vi "MainNR.vi"(10 "JQMHStartup":refnum<class "RQMHStartup.lvclass">, 11 "NewTemplate in":refnum<class "Shell.lvclass">) -> ()   [LabVIEW 2024, in "Shell.lvclass"]
uses:
  Shell.lvclass
  RQMHCore/Startup/RQMHStartup.lvclass
  RQMHCore/ModQueue/RQMHMessageQueue.lvclass/RQMHMessageQueue.ctl
  RQMHCore/ModuleCore/InitialiseReplyArgs.ctl
  RQMHCore/ModuleCore/RQMHModule.lvclass/RQMHModule.ctl
  Do Something ReplyArgs.ctl
  Do Something Args.ctl
  GetContents ReplyArgs.ctl
  Maximise Args.ctl
  RQMHCore/ModuleCore/Read ModuleName.vi
  RQMHCore/ModuleCore/Read External Start.vi
  RQMHCore/ModQueue/Delacor_lib_QMH_Enqueue Message (Single).vi
  RQMHCore/ModQueue/RQMHMessageQueue.lvclass
  RQMHCore/ModuleCore/RQMHModule.lvclass
  RQMHCore/Shared/RQMHShared.lvlib
panel:
  out "error out":errorcluster
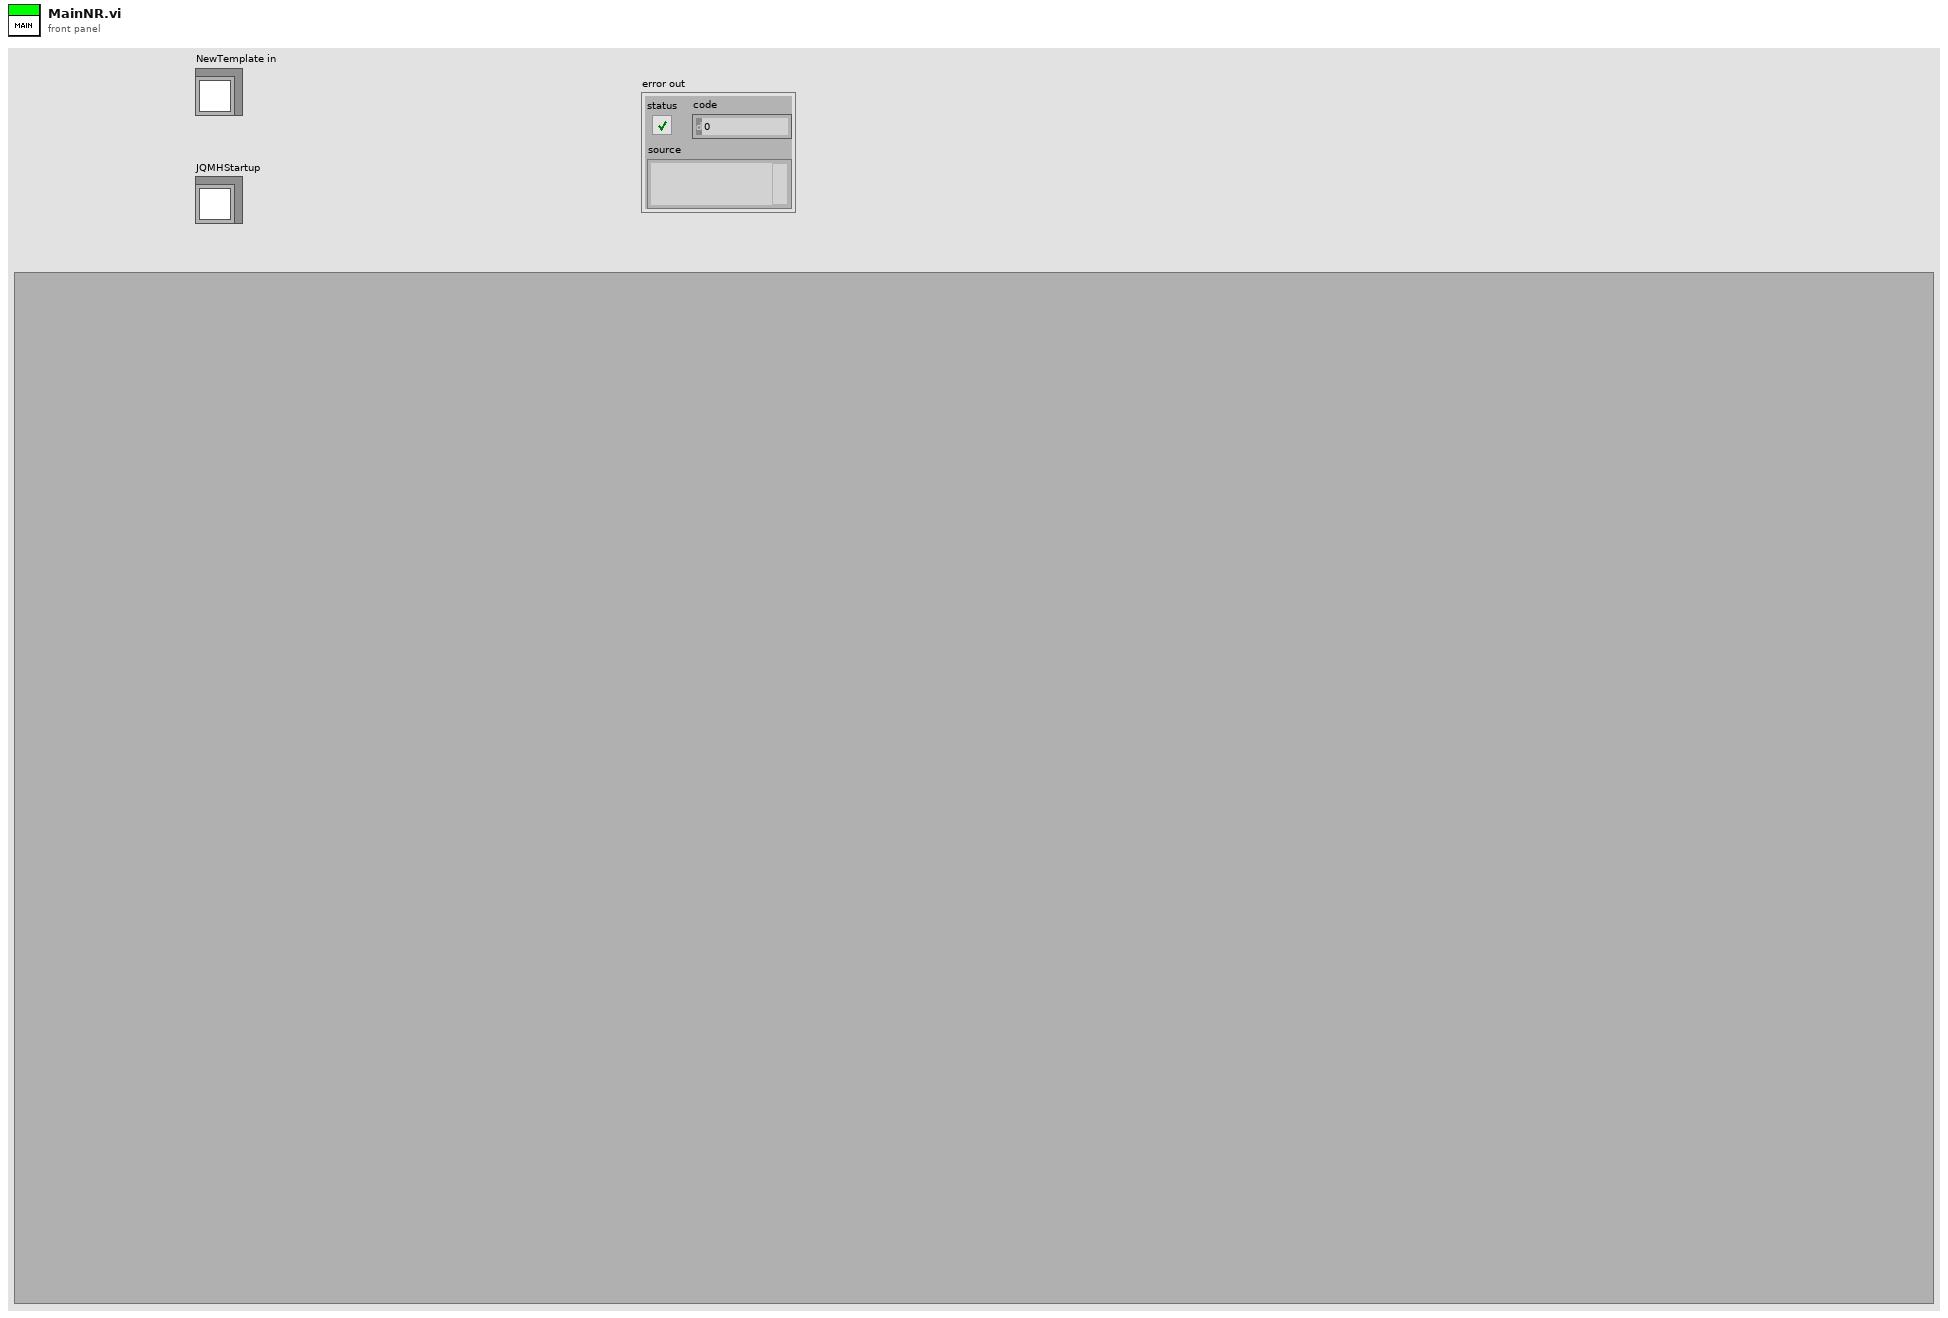
[diagram p1: front panel]
types:
  T1 = typedef "Shell.lvclass/Request Events--cluster.ctl" = cluster{"Do Something":refnum<user-event>, "GetContents":refnum<user-event>, "Maximise":refnum<user-event>, "Minimise":refnum<user-event>}
  T2 = cluster{"Stop Module":refnum<user-event>, "Requests":T1}
  T3 = enum32{"Invalid", "Standard", "Closed", "Hidden", "Minimized", "Maximized"}
  T4 = typedef "RQMHModule.lvclass/InitialiseReplyArgs.ctl" = cluster{"Did Init?":bool}
  T5 = typedef "Shell.lvclass/Do Something Args.ctl" = cluster{"Msg":string}
  T6 = typedef "Shell.lvclass/Do Something ReplyArgs.ctl" = cluster{"Value":dbl, "Boolean":bool}
  T7 = typedef "Shell.lvclass/GetContents ReplyArgs.ctl" = cluster{"Sub Panel":refnum<vi>}
  T8 = typedef "Shell.lvclass/Maximise Args.ctl" = cluster{"Maximise":bool}
  T9 = typedef "RQMHModule.lvclass/Reply.ctl" = cluster{"Expects Reply":bool, "Reply":refnum<notifier>}
  T10 = typedef "Shell.lvclass/GetContents Args.ctl" = cluster{"String":string}
  T11 = typedef "Shell.lvclass/Minimise Args.ctl" = cluster{"null":bool}
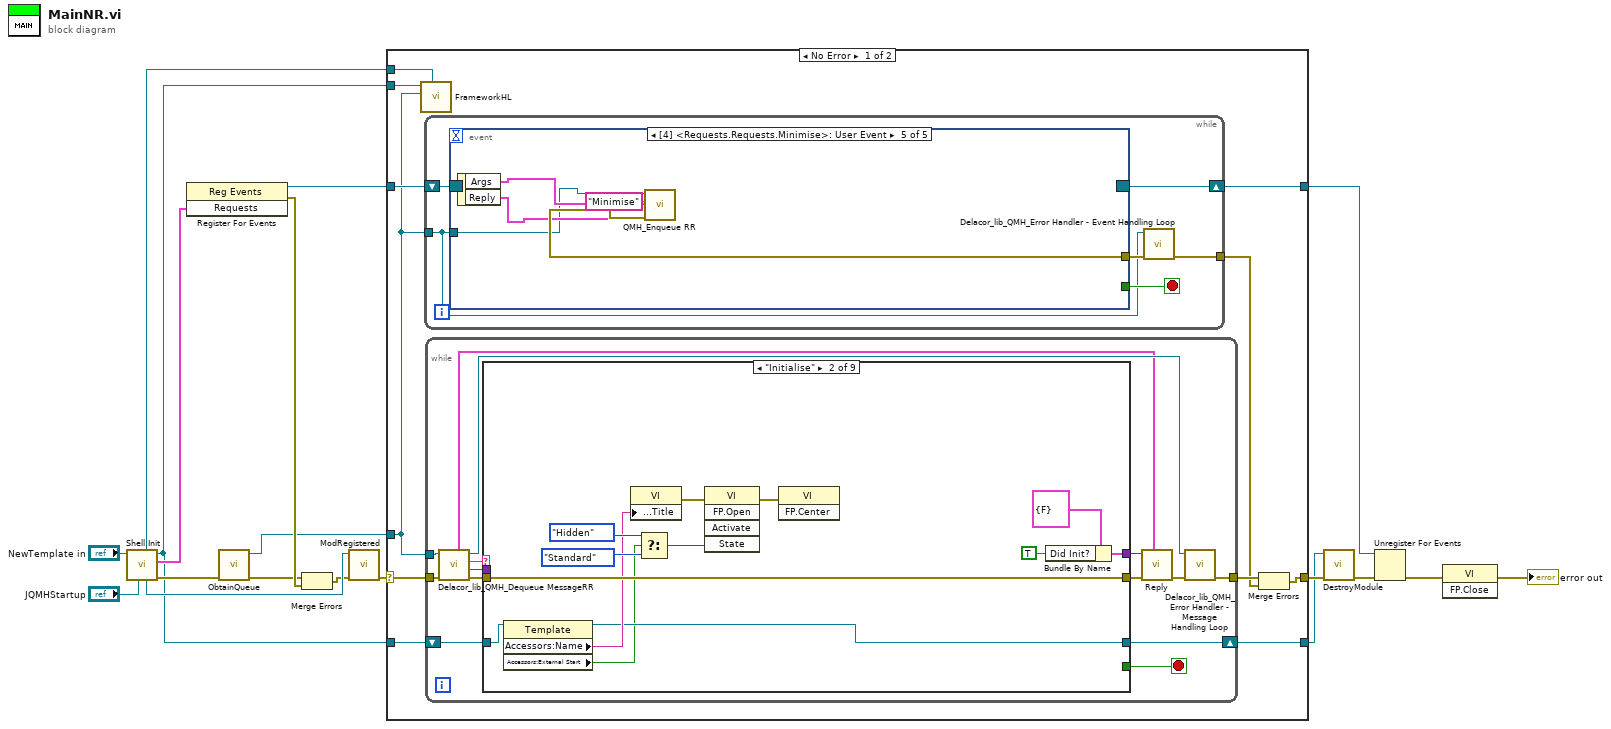
[diagram p0: block diagram]
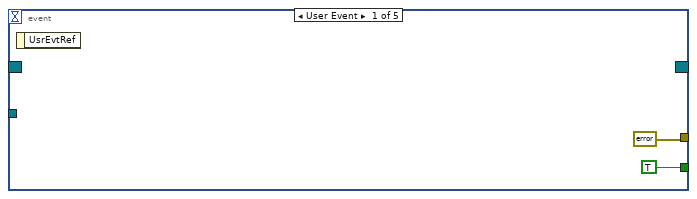
[diagram p2: hidden frame]
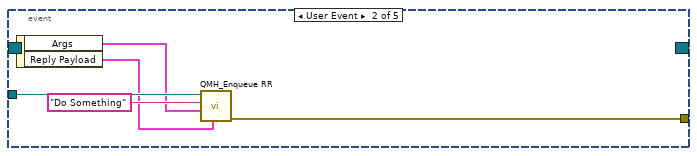
[diagram p3: hidden frame]
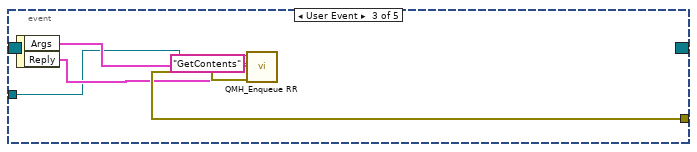
[diagram p4: hidden frame]
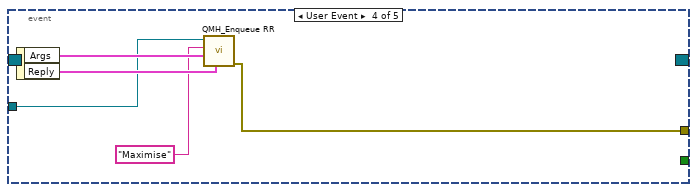
[diagram p5: hidden frame]
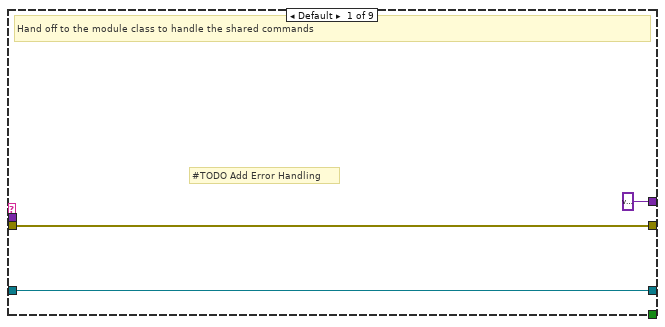
[diagram p6: hidden frame]
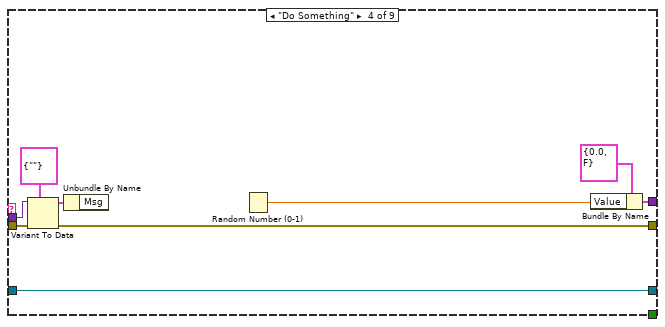
[diagram p8: hidden frame]
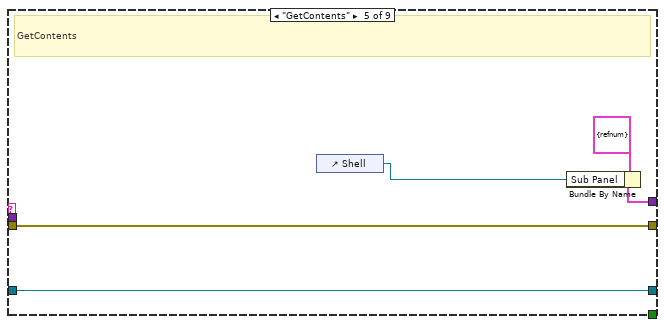
[diagram p9: hidden frame]
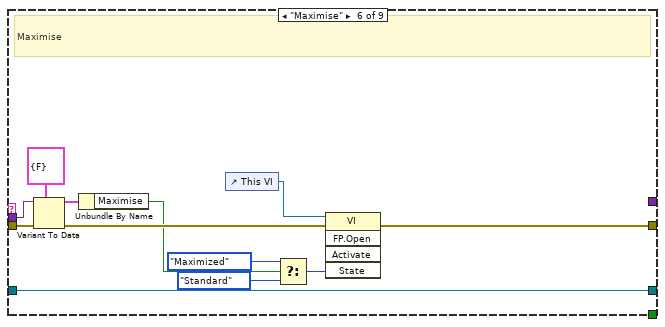
[diagram p10: hidden frame]
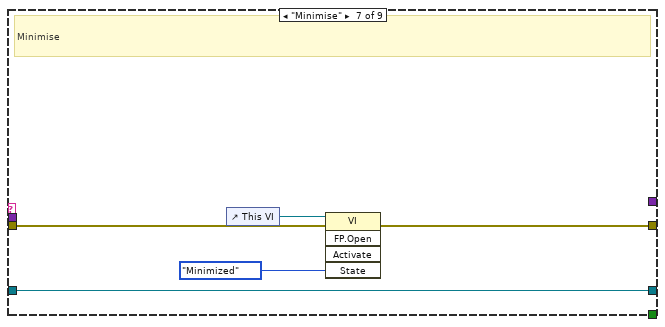
[diagram p11: hidden frame]
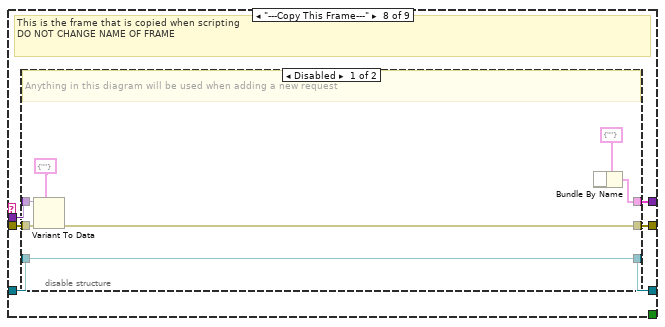
[diagram p12: hidden frame]
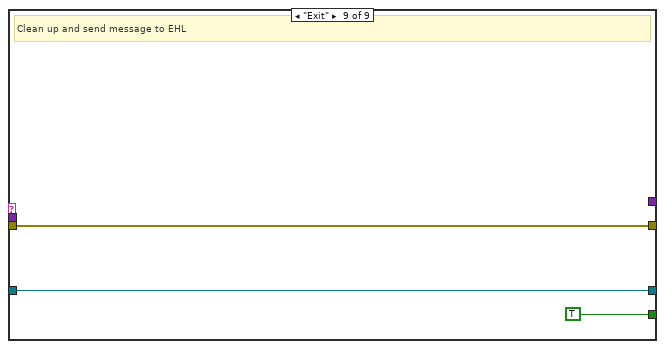
[diagram p14: hidden frame]
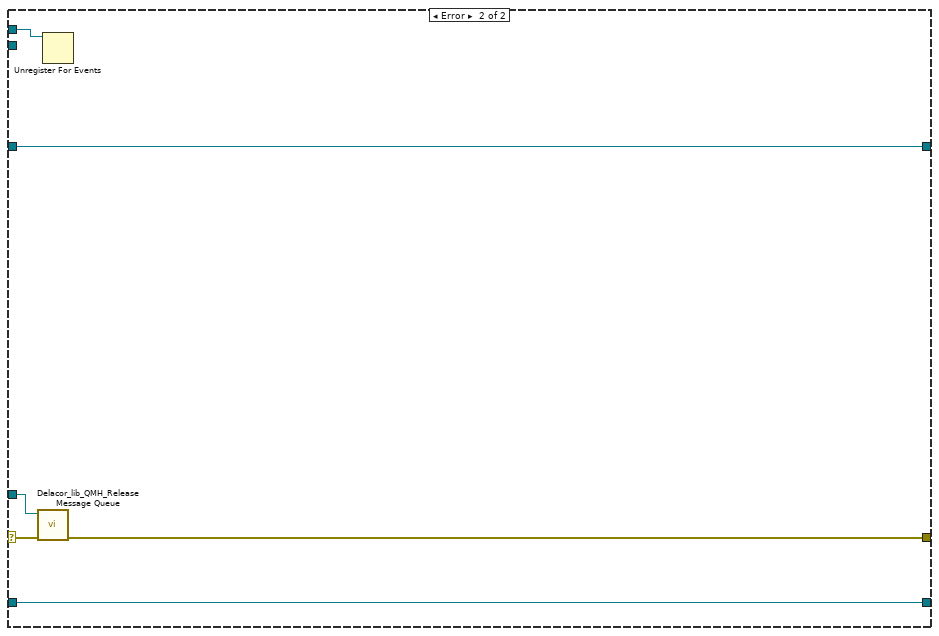
[diagram p15: hidden frame]
diagram:
  n1 = call "Shell.Init.vi"("JQMHStartup in"="JQMHStartup", "NewTemplate in"="NewTemplate in") -> ("error out"=w13:errorcluster, "Requests"=w4:T2, "NewTemplate out"=w3:refnum<class "Shell.lvclass">, "JQMHStartup out"=w11:refnum<class "RQMHStartup.lvclass">, "StandardRequests"=w7:refnum<event-registration>)  [unwired: 4 in, 1 out]
  n2 = register-events(w4) -> (reference out=w6:refnum<event-registration>, error out=w19:errorcluster)  [unwired: 2 in]
  n3 = call "ObtainQueue.vi"("error in"=w13) -> ("error out"=w12:errorcluster, "Message Queue"=w8:refnum<class "RQMHMessageQueue.lvclass">)  [unwired: 9 in]
  n4 = Merge Errors(w12, w19) -> (w9:errorcluster)
  n5 = call "ModRegistered.vi"("error in (no error)"=w9, "JQMHStartup in"=w11) -> ("error out"=w10:errorcluster)  [unwired: 9 in]
  n6 = case "RQMH_MAIN" shown="No Error" w10 {
    selector: w10 -> [w27 w143]
    tunnel: w3 -> [w30 w142]
    tunnel: [w29 w145] -> w18
    tunnel: w6 -> [w28 w145]
    tunnel: w8 -> [w21 w144]
    tunnel: [w26 w142] -> w5
    tunnel: [w23 w141] -> w15
    tunnel: w3 -> [w22 _]
    tunnel: w7 -> [w20 w140]
    frame No Error {
      n7 = call-dynamic "FrameworkHL.vi"("StandardRequests"=w20, "Message Queue"=w21, "JQMHModule in"=w22) -> ()  [unwired: 9 in]
      n8 = while {
        shift-right: [w36] -> w29
        shift-left: w28 -> [w31]
        tunnel: w21 -> [w32]
        tunnel: [w33] -> w24
        stop <- w35 stop-if-true
        n9 = event "RQMH_EVENT_MAIN" shown="[4] <Requests.Requests.Minimise>: User Event" {
          selector: w31 -> [_ _ _ _ _]
          dyn-events: [_ _ _ _ _] -> w36
          timeout: _ -> [_ _ _ _ _]
          tunnel: [TRUE _ _ _ _] -> w35
          tunnel: w32 -> [_ w43 w45 w50 w55]
          tunnel: [errorcluster {"status"=FALSE, "code"=0, "source"=""} ("error out") w40 w48 w53 w58] -> w34
          event User Event {
            n10 = event-data() -> ()  [unwired: 1 in, 1 out]
          }
          event User Event {
            n11 = event-data() -> ("Args"=w41:T5, "Reply Payload"=w39:T9)  [unwired: 1 in]
            n12 = call "QMH_Enqueue RR.vi"("Reply"=w39, "Message Data"=w41, "Message"="Do Something", "Message Queue in"=w43) -> ("error out"=w40:errorcluster)  [unwired: 6 in, 1 out]
          }
          event User Event {
            n13 = event-data() -> ("Args"=w46:T10, "Reply"=w47:T9)  [unwired: 1 in]
            n14 = call "QMH_Enqueue RR.vi"("Reply"=w47, "Message Data"=w46, "Message"="GetContents", "Message Queue in"=w45) -> ("error out"=w48:errorcluster)  [unwired: 6 in, 1 out]
          }
          event User Event {
            n15 = event-data() -> ("Args"=w51:T8, "Reply"=w52:T9)  [unwired: 1 in]
            n16 = call "QMH_Enqueue RR.vi"("Reply"=w52, "Message Data"=w51, "Message"="Maximise", "Message Queue in"=w50) -> ("error out"=w53:errorcluster)  [unwired: 6 in, 1 out]
          }
          event User Event {
            n17 = event-data() -> ("Args"=w56:T11, "Reply"=w57:T9)  [unwired: 1 in]
            n18 = call "QMH_Enqueue RR.vi"("Reply"=w57, "Message Data"=w56, "Message"="Minimise", "Message Queue in"=w55) -> ("error out"=w58:errorcluster)  [unwired: 6 in, 1 out]
          }
        }
        n19 = call-dynamic "Delacor_lib_QMH_Error Handler - Event Handling Loop.vi"("error in"=w34, "Message Queue in"=w32) -> ("dup error in"=w33:errorcluster)  [unwired: 8 in, 1 out]
      }
      n20 = while {
        tunnel: w21 -> [w67]
        tunnel: w27 -> [w66]
        shift-right: [w69] -> w26
        shift-left: w30 -> [w70]
        tunnel: [w68] -> w25
        stop <- w72 stop-if-true
        n21 = call-dynamic "Delacor_lib_QMH_Dequeue MessageRR.vi"("error in"=w66, "Message Queue in"=w67) -> ("error out"=w65:errorcluster, "Message Data"=w63:variant, "Message"=w64:string, "Message Queue out"=w71:refnum<class "RQMHMessageQueue.lvclass">, "Reply"=w59:T9)  [unwired: 5 in]
        n22 = case "RQMH_MESSAGE_CASES" shown="\"Initialise\"" w64 {
          tunnel: [_ _ _ _ _ _ _ _ TRUE] -> w72
          tunnel: w70 -> [w74 w77 w89 w99 w103 w115 w121 w125 w138]
          tunnel: w63 -> [_ _ _ w95 _ w114 _ w123 _]
          tunnel: w65 -> [w75 w88 w90 w94 w104 w116 w119 w127 w137]
          tunnel: [w75 w88 w90 w93 w104 w109 w118 w126 w137] -> w62
          tunnel: [w74 w78 w89 w99 w103 w115 w121 w124 w138] -> w69
          tunnel: [variant w87 _ w98 w102 _ _ w122 _] -> w60
          frame Default {
            # "#TODO Add Error Handling"
            # "Hand off to the module class to handle the shared commands"
          }
          frame "Initialise" {
            n23 = property class="Template"(reference=w77) -> (reference out=w78:refnum<class "Shell.lvclass">, "Accessors:Name"=w79:string, "Accessors:External Start"=w76:bool)  [unwired: 1 in, 1 out]
            n24 = property on="Property Node" class="VI"("Front Panel.Title"=w79) -> (error out=w85:errorcluster)  [unwired: 2 in, 1 out]
            n25 = Select(t=T3."Hidden" ("State"), s=w76, f=T3."Standard" ("State")) -> (s? t:f=w81:T3)
            n26 = invoke on="Invoke Node" class="VI" method="FP.Open"(error in=w85, "State"=w81) -> (error out=w84:errorcluster)  [unwired: 3 in, 4 out]
            n27 = invoke on="Invoke Node" class="VI" method="FP.Center"(error in=w84) -> ()  [unwired: 2 in, 3 out]
            n28 = Bundle By Name(cluster=T4 {"Did Init?"=FALSE} ("Args"), "Did Init?"=TRUE) -> (w87:T4)
          }
          frame "---Module Specific---" {
          }
          frame "Do Something" {
            n29 = Variant To Data(error in=w94, type=T5 {"Msg"=""} ("Do Something Args"), Variant=w95) -> (data=w91:T5, error out=w93:errorcluster)
            n30 = Unbundle By Name(w91) -> ()  [unwired: 1 out]
            n31 = Random Number (0-1)() -> (number: 0 to 1=w96:dbl)
            n32 = Bundle By Name(cluster=T6 {"Value"=0.0, "Boolean"=FALSE}, "Value"=w96) -> (w98:T6)
          }
          frame "GetContents" {
            # "GetContents"
            n33 = control-ref of="Shell"() -> (w100:refnum<vi>)
            n34 = Bundle By Name(cluster=T7 {"Sub Panel"=refnum} ("RQMH_MHL_REPLY_PL"), "Sub Panel"=w100) -> (w102:T7)
          }
          frame "Maximise" {
            # "Maximise"
            n35 = Variant To Data(error in=w116, type=T8 {"Maximise"=FALSE} ("RQMH_MHL_MSG_PL"), Variant=w114) -> (data=w112:T8, error out=w110:errorcluster)
            n36 = Unbundle By Name(w112) -> ("Maximise"=w107:bool)
            n37 = control-ref of="This VI"() -> (w111:refnum<vi>)
            n38 = Select(t=T3."Maximized" ("State"), s=w107, f=T3."Standard" ("State")) -> (s? t:f=w105:T3)
            n39 = invoke class="VI" method="FP.Open"(reference=w111, error in=w110, "State"=w105) -> (error out=w109:errorcluster)  [unwired: 2 in, 4 out]
          }
          frame "Minimise" {
            # "Minimise"
            n40 = control-ref of="This VI"() -> (w120:refnum<vi>)
            n41 = invoke class="VI" method="FP.Open"(reference=w120, error in=w119, "State"=T3."Minimized") -> (error out=w118:errorcluster)  [unwired: 2 in, 4 out]
          }
          frame "---Copy This Frame---" {
            # "This is the frame that is copied when scripting\nDO NOT CHANGE NAME OF FRAME"
            n42 = disable-structure shown="Disabled" {
              disable-tunnel: w127 -> [w131 w136]
              disable-tunnel: [w132 w136] -> w126
              disable-tunnel: w125 -> [w134 w135]
              disable-tunnel: [w134 w135] -> w124
              disable-tunnel: w123 -> [w133 _]
              disable-tunnel: [w129 _] -> w122
              frame Disabled {
                # "Anything in this diagram will be used when adding a new request"
                n43 = Variant To Data(error in=w131, type=cluster{string} {""} ("RQMH_MHL_MSG_PL"), Variant=w133) -> (error out=w132:errorcluster)  [unwired: 1 out]
                n44 = Bundle By Name(cluster=cluster{string} {""} ("RQMH_MHL_REPLY_PL")) -> (w129:cluster{string})  [unwired: 1 in]
              }
              frame Enabled {
              }
            }
          }
          frame "Exit" {
            # "Clean up and send message to EHL"
          }
        }
        n45 = call "Reply.vi"("Reply"=w59, "error in (no error)"=w62, "ReplyPayload"=w60) -> ("error out"=w61:errorcluster)  [unwired: 8 in]
        n46 = call-dynamic "Delacor_lib_QMH_Error Handler - Message Handling Loop.vi"("error in"=w61, "Message Queue in"=w71) -> ("dup error in"=w68:errorcluster)  [unwired: 8 in, 1 out]
      }
      n47 = Merge Errors(w25, w24) -> (w23:errorcluster)
    }
    frame Error {
      n48 = call-dynamic "Delacor_lib_QMH_Release Message Queue.vi"("error in"=w143, "Message Queue"=w144) -> ("error out"=w141:errorcluster)  [unwired: 9 in]
      n49 = Unregister For Events(event registration refnum=w140) -> ()  [unwired: 1 in, 1 out]
    }
  }
  n50 = call "DestroyModule.vi"("error in (no error)"=w15, "JQMHModule in"=w5) -> ("error out"=w17:errorcluster)  [unwired: 9 in]
  n51 = Unregister For Events(event registration refnum=w18, error in=w17) -> (error out=w2:errorcluster)
  n52 = invoke class="VI" method="FP.Close"(error in=w2) -> (error out=→"error out":errorcluster)  [unwired: 2 in, 2 out]
